vi "ResetSession.vi"(7 "Python in":T1, 8 "error in":errorcluster, 11 "Arduino in":T3) -> (0 "error out":errorcluster, 3 "Python out":T1)   [LabVIEW 2022 SP3]
uses:
  PythonCtrl.ctl
  Processors.ctl
  ArduinoCtrl.ctl
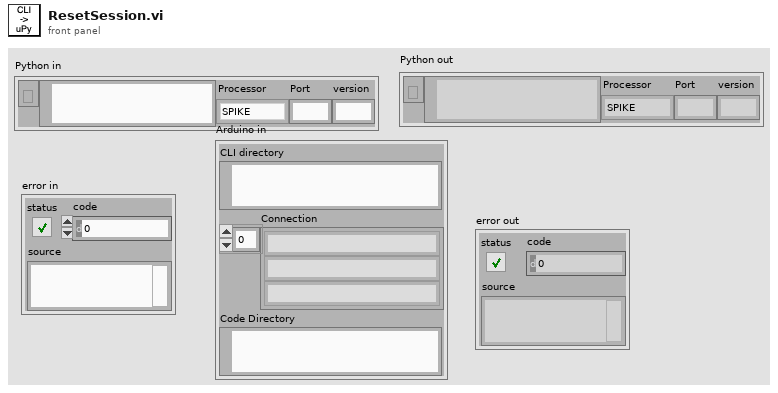
[diagram p1: front panel]
types:
  T1 = typedef "PythonCtrl.ctl" = cluster{"session":refnum<k35>, "PyPath":path, "Processor":T2, "Port":string, "version":string}
  T2 = typedef "Processors.ctl" = enum16{"SPIKE", "Pi", "Pi_ssh", "OpenMV", "Dunio"}
  T3 = typedef "ArduinoCtrl.ctl" = cluster{"CLI directory":path, "Connection":string[], "Code Directory":path}
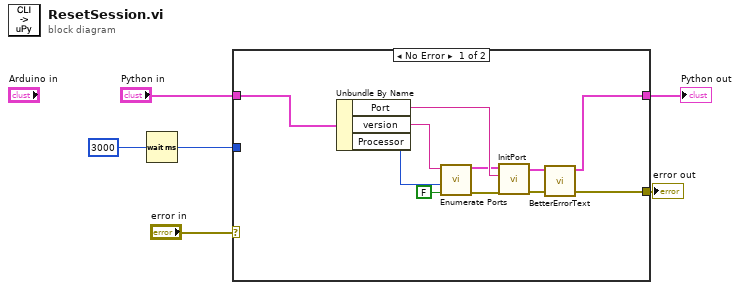
[diagram p0: block diagram]
diagram:
  n1 = Wait (ms)(milliseconds to wait=u32 3000) -> (millisecond timer value=w3:u32)
  n2 = case shown="No Error" "error in" {
    selector: "error in" -> [_ w18]
    tunnel: [w9 w18] -> w6
    tunnel: w3 -> [_ _]
    tunnel: [w8 w17] -> w2
    tunnel: "Python in" -> [w7 w17]
    frame No Error {
      n3 = Unbundle By Name(w7) -> ("Port"=w16:string, "version"=w12:string, "Processor"=w11:T2)
      n4 = call "Enumerate Ports.vi"("list?"=FALSE, "Processor"=w11, "Python version"=w12) -> ("error out"=w13:errorcluster, "Python"=w14:T1)  [unwired: 3 in, 4 out]
      n5 = call "InitPort.vi"("error in (no error)"=w13, "Port"=w16, "Python"=w14) -> ("error out"=w9:errorcluster, "Python out"=w10:T1)  [unwired: 6 in, 1 out]
      n6 = call "BetterErrorText.vi"("error in (no error)"=w9, "Python"=w10) -> ("Python out"=w8:T1)  [unwired: 8 in, 1 out]
    }
    frame Error {
    }
  }
  "error out" <- w6
  "Python out" <- w2
